vi "CheckParams.vi"(10 "FPGA CLUSTER":T1={"Start freq. [Hz]"=10.0, "Sweep duration [s]"=0.1, "Freq. step [Hz]"=0.1, "DAC Sample Rate"=1388888.8888, "ADC Sample Rate"=50000000.0, "CMD port"=2047, "DFAST port"=2048, "CMD ID"=refnum, "DFAST ID"=refnum, "CMD error out"={"status"=FALSE, "code"=0, "source"=""}, "FPGA IP"="192.168.1.12", "DFAST error out "={"status"=FALSE, "code"=0, "source"=""}, "Stop freq. [Hz]"=0.0, "Discrete sweep"=FALSE, "Initial NCO"=10, "Difference NCO"=0, "step NCO"=0, "Final NCO"=0, "clocks for step"=0, "demodulation"=FALSE, "NCO Phase Precision"=32, "NCO Sample Rate"=50000000.0, "Time for step [s]"=0.1, "NCO freq. resolution"=32.0, "Sweep speed [Hz/s]"=0.1, "Connected"=FALSE, "Slew Rate [V/us]"=50000000.0, "Parameters_ok"=FALSE, "Amplitude [mVpp]"=10.0, "Scale Factor"=0.999969482421875, "Acquiring"=FALSE, "DAC-ADC Latency"=1, "Digital Gain"=0, "Number of steps"=1, "Averaging preferred"=FALSE, "Filter Order"=1, "Settling"=enum."99,9%"} {"Filter Order" min=1 max=4; "Number of steps" min=1; "Digital Gain" items=["1", "2", "4", "8", "16", "32", "64"]; "DAC-ADC Latency" min=1 format="%#_4g"; "Amplitude [mVpp]" min=4.0 max=200.0 format="%.3f"; "Sweep speed [Hz/s]" min=0.001 max=5.0 step=0.001 format="%.3f"; "Time for step [s]" min=0.001 max=5.0 step=0.001 format="%.3f"; "clocks for step" min=1 max=5 step=1; "Final NCO" min=4 max=200; "step NCO" min=1 max=5 step=1; "Difference NCO" min=1 max=5 step=1; "Initial NCO" min=4 max=200; "Stop freq. [Hz]" min=4.0 max=200.0 format="%.3f"; "Freq. step [Hz]" min=0.001 max=5.0 step=0.001 format="%.3f"; "Sweep duration [s]" min=0.001 max=5.0 step=0.001 format="%.3f"; "Start freq. [Hz]" min=4.0 max=200.0 format="%.3f"}, 11 "FPGA in":refnum<queue>) -> (2 "Not Valid":bool, 3 "FPGA out":refnum<queue>)   [LabVIEW 2019, in "FPGA.lvlib"]
uses:
  FPGA.lvlib
  FPGA.ctl
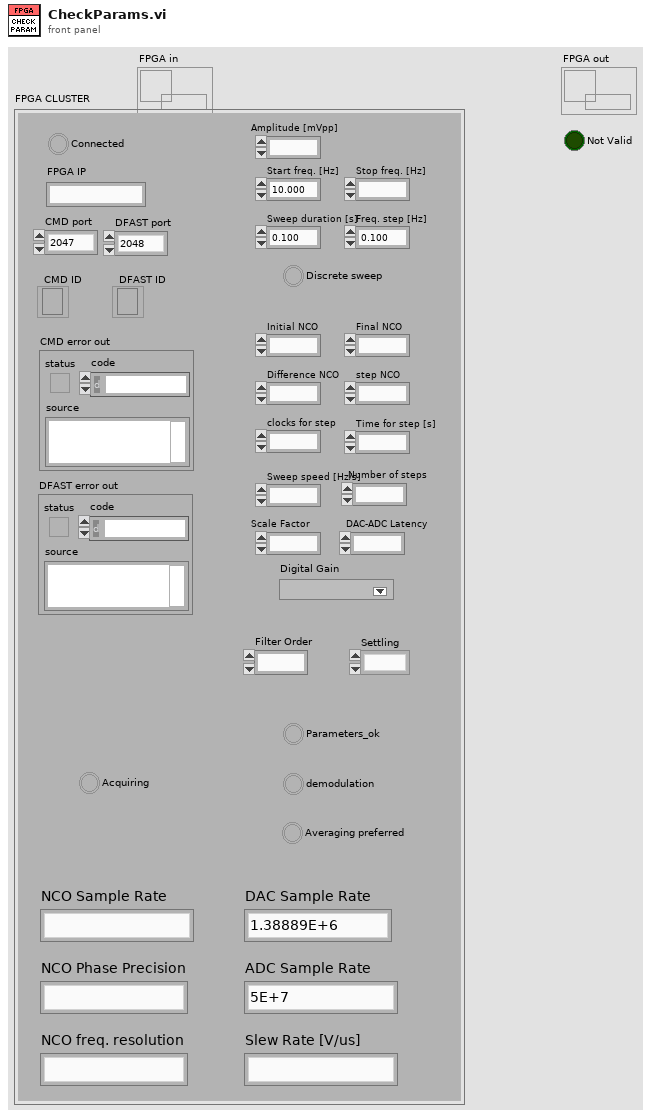
[diagram p1: front panel]
types:
  T1 = typedef "FPGA.lvlib/FPGA.ctl" = cluster{"Start freq. [Hz]":dbl, "Sweep duration [s]":dbl, "Freq. step [Hz]":dbl, "DAC Sample Rate":dbl, "ADC Sample Rate":dbl, "CMD port":u16, "DFAST port":u16, "CMD ID":refnum<k16>, "DFAST ID":refnum<k16>, "CMD error out":errorcluster, "FPGA IP":string, "DFAST error out ":errorcluster, "Stop freq. [Hz]":dbl, "Discrete sweep":bool, "Initial NCO":u32, "Difference NCO":i32, "step NCO":i64, "Final NCO":u32, "clocks for step":u32, "demodulation":bool, "NCO Phase Precision":u32, "NCO Sample Rate":dbl, "Time for step [s]":dbl, "NCO freq. resolution":dbl, "Sweep speed [Hz/s]":dbl, "Connected":bool, "Slew Rate [V/us]":dbl, "Parameters_ok":bool, "Amplitude [mVpp]":dbl, "Scale Factor":fxp<+,16,0>, "Acquiring":bool, "DAC-ADC Latency":u16, "Digital Gain":i32, "Number of steps":i32, "Averaging preferred":bool, "Filter Order":u32, "Settling":enum16{"99%", "99,9%"}}
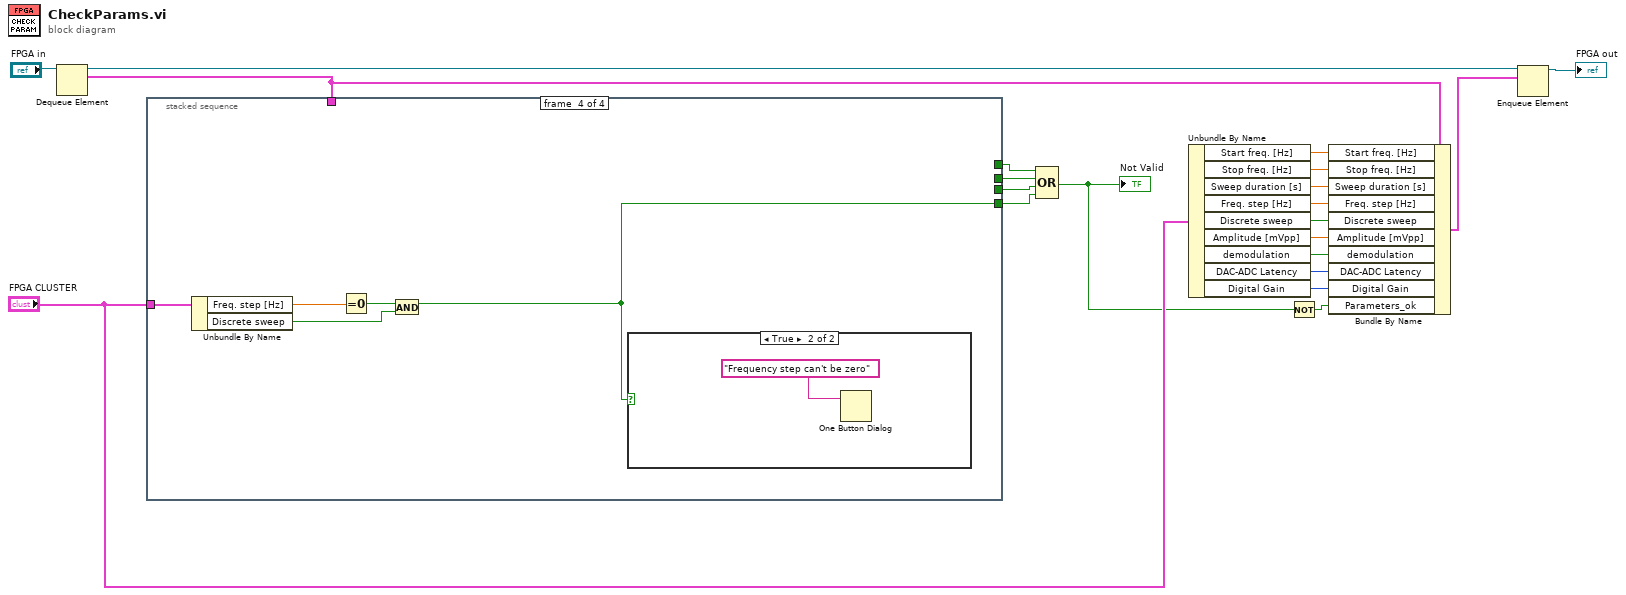
[diagram p0: block diagram]
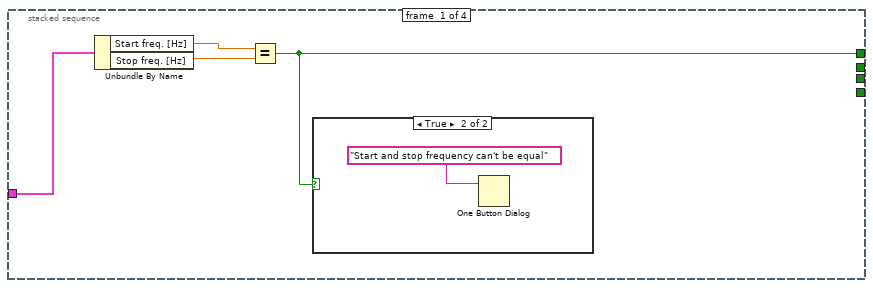
[diagram p2: hidden frame]
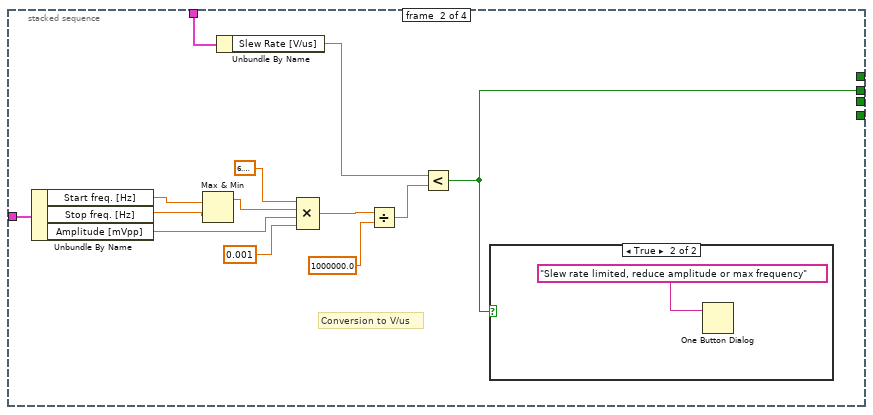
[diagram p4: hidden frame]
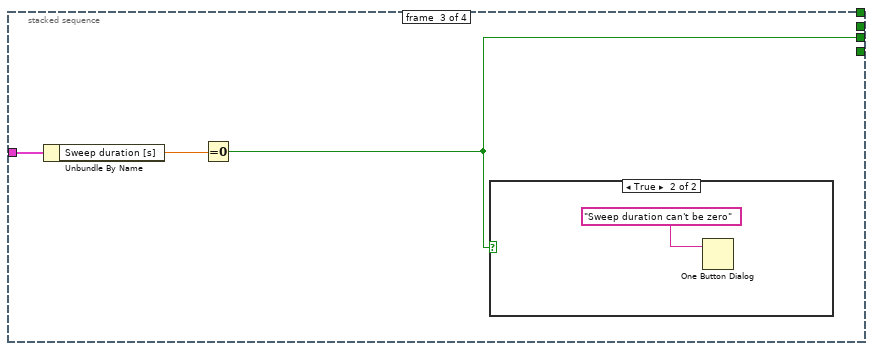
[diagram p6: hidden frame]
diagram:
  n1 = Dequeue Element(queue="FPGA in") -> (queue out=w19:refnum<queue>, element=w16:T1)  [unwired: 2 in, 2 out]
  n2 = stacked-sequence {
    tunnel: "FPGA CLUSTER" -> [w22 w39 w43 w49]
    tunnel: [w23 _ _ _] -> w18
    tunnel: w16 -> [_ w30 _ _]
    tunnel: [_ w27 _ _] -> w17
    tunnel: [_ _ w41 _] -> w13
    tunnel: [_ _ _ w46] -> w12
    frame #0 {
      n3 = Unbundle By Name(w22) -> ("Start freq. [Hz]"=w25:dbl, "Stop freq. [Hz]"=w24:dbl)
      n4 = Equal?(x=w25, y=w24) -> (x = y?=w23:bool)
      n5 = case shown="True" w23 {
        frame False {
        }
        frame True {
          n6 = One Button Dialog(message="Start and stop frequency can't be equal") -> ()  [unwired: 1 in, 1 out]
        }
      }
    }
    frame #1 {
      # "Conversion to V/us"
      n7 = Unbundle By Name(w39) -> ("Start freq. [Hz]"=w38:dbl, "Stop freq. [Hz]"=w37:dbl, "Amplitude [mVpp]"=w34:dbl)
      n8 = Max & Min(x=w38, y=w37) -> (max(x,y)=w36:dbl)  [unwired: 1 out]
      n9 = Unbundle By Name(w30) -> ("Slew Rate [V/us]"=w29:dbl)
      n10 = Compound Arithmetic op=MULTIPLY(6.283185307179586, w36, w34, 0.001 ("value")) -> (w32:dbl)
      n11 = Divide(x=w32, y=1000000.0) -> (x/y=w28:dbl)
      n12 = Less?(x=w29, y=w28) -> (x < y?=w27:bool)
      n13 = case shown="True" w27 {
        frame False {
        }
        frame True {
          n14 = One Button Dialog(message="Slew rate limited, reduce amplitude or max frequency") -> ()  [unwired: 1 in, 1 out]
        }
      }
    }
    frame #2 {
      n15 = Unbundle By Name(w43) -> ("Sweep duration [s]"=w42:dbl)
      n16 = Equal To 0?(x=w42) -> (x = 0?=w41:bool)
      n17 = case shown="True" w41 {
        frame False {
        }
        frame True {
          n18 = One Button Dialog(message="Sweep duration can't be zero") -> ()  [unwired: 1 in, 1 out]
        }
      }
    }
    frame #3 {
      n19 = Unbundle By Name(w49) -> ("Freq. step [Hz]"=w48:dbl, "Discrete sweep"=w45:bool)
      n20 = Equal To 0?(x=w48) -> (x = 0?=w47:bool)
      n21 = And(x=w47, y=w45) -> (x .and. y?=w46:bool)
      n22 = case shown="True" w46 {
        frame False {
        }
        frame True {
          n23 = One Button Dialog(message="Frequency step can't be zero") -> ()  [unwired: 1 in, 1 out]
        }
      }
    }
  }
  n24 = Compound Arithmetic op=OR(w18, w17, w13, w12) -> (w1:bool)
  "Not Valid" <- w1
  n25 = Unbundle By Name("FPGA CLUSTER") -> ("Start freq. [Hz]"=w9:dbl, "Stop freq. [Hz]"=w8:dbl, "Sweep duration [s]"=w7:dbl, "Freq. step [Hz]"=w11:dbl, "Discrete sweep"=w10:bool, "Amplitude [mVpp]"=w6:dbl, "demodulation"=w5:bool, "DAC-ADC Latency"=w4:u16, "Digital Gain"=w3:i32)
  n26 = Not(x=w1) -> (.not. x?=w2:bool)
  n27 = Bundle By Name(cluster=w16, "Start freq. [Hz]"=w9, "Stop freq. [Hz]"=w8, "Sweep duration [s]"=w7, "Freq. step [Hz]"=w11, "Discrete sweep"=w10, "Amplitude [mVpp]"=w6, "demodulation"=w5, "DAC-ADC Latency"=w4, "Digital Gain"=w3, "Parameters_ok"=w2) -> (w14:T1)
  n28 = Enqueue Element(queue=w19, element=w14) -> (queue out=→"FPGA out":refnum<queue>)  [unwired: 2 in, 2 out]
